vi "Configure Math Rolling Average.vi"(0 "VISA resource name":refnum<visa-resource-name>, 1 "Count (1)":i32=1 min=1 max=1500, 5 "Channel (001)":string="001", 7 "Enable Rolling Average (False)":bool, 9 "Interval (6: 10s)":u16(ring)=6 items=["1s", "2s", "3s", "4s", "5s", "6s", "10s", "12s", "15s", "20s", "30s", "1min", "2min", "3min", "4min", "5min", "6min", "10min", "12min", "15min", "20min", "30min", "1h"], 11 "error in (no error)":errorcluster) -> (4 "VISA resource name out":refnum<visa-resource-name>, 6 "Channel":string, 15 "error out":errorcluster)   [LabVIEW 2020, in "Yokogawa GX Series.lvlib"]
doc: "Sets rolling average on a math channel.\n\nCommand: SRolAveMath"
uses:
  <instrlib>/Yokogawa GX Series/Yokogawa GX Series.lvlib
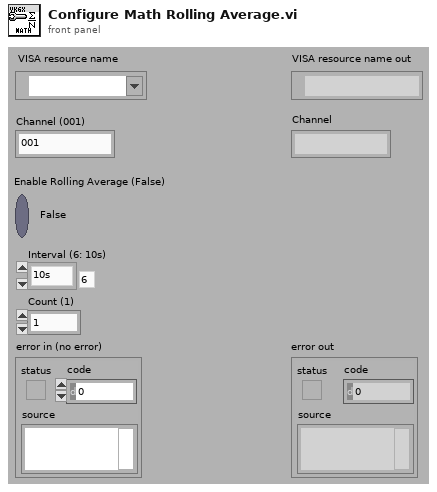
[diagram p1: front panel]
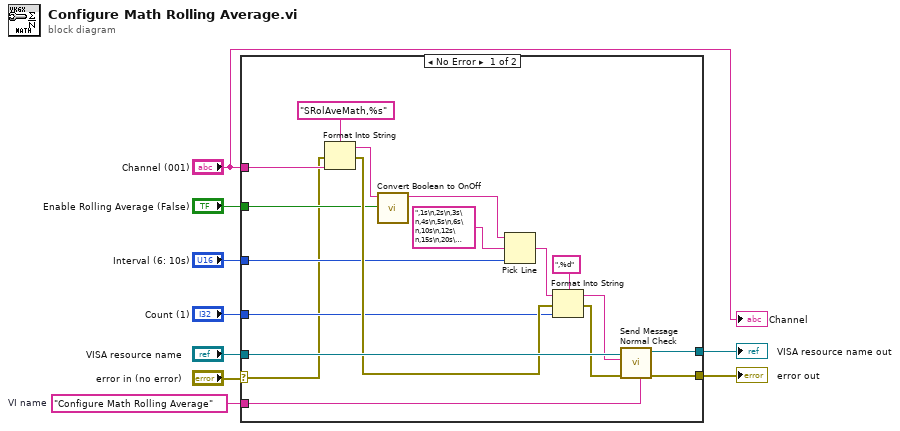
[diagram p0: block diagram]
diagram:
  w8 = "Configure Math Rolling Average"  # VI name
  n1 = case shown="No Error" "error in (no error)" {
    selector: "error in (no error)" -> [w10 w28]
    tunnel: "VISA resource name" -> [w27 w29]
    tunnel: w8 -> [w26 _]
    tunnel: [w25 w29] -> w7
    tunnel: [w24 w28] -> w6
    tunnel: "Count (1)" -> [w18 _]
    tunnel: "Interval (6: 10s)" -> [w17 _]
    tunnel: "Channel (001)" -> [w12 _]
    tunnel: "Enable Rolling Average (False)" -> [w11 _]
    frame No Error {
      n2 = Format Into String(format string="SRolAveMath,%s", error in=w10, w12) -> (resulting string=w14:string, error out=w21:errorcluster)  [unwired: 1 in]
      n3 = call <instrlib>:"Convert Boolean to OnOff.vi"("On/Off"=w11, "Initial String (\"\")"=w14) -> ("Resulting String"=w13:string)  [unwired: 9 in]
      n4 = Pick Line(string ("")=w13, multi-line string=",1s\n,2s\n,3s\n,4s\n,5s\n,6s\n,10s\n,12s\n,15s\n,20s\n,30s\n,1min\n,2min\n,3min\n,4min\n,5min\n,6min\n,10min\n,12min\n,15min\n,20min\n,30min\n,1h", line index=w17) -> (output string=w16:string)
      n5 = Format Into String(format string=",%d", initial string=w16, error in=w21, w18) -> (resulting string=w20:string, error out=w19:errorcluster)
      n6 = call <instrlib>:"Send Message Normal Check.vi"("Source (\"\")"=w26, "error in (no error)"=w19, "Send Message (\"\")"=w20, "VISA resource name"=w27) -> ("error out"=w24:errorcluster, "VISA resource name out"=w25:refnum<visa-resource-name>)  [unwired: 2 in, 4 out]
    }
    frame Error {
    }
  }
  "error out" <- w6
  "VISA resource name out" <- w7
  "Channel" <- "Channel (001)"
